vi "GUI Manual.vi"() -> ()   [LabVIEW 2019]
panel:
  in  "String 3":string="Блок управление ВБ"
  in  "String 2":string="Гидростанция очистки и охлаждения"
  in  "Tab Control 2":enum32{"Управление", "Настройки"}(tab)
  out "DI 31":bool caption="Релеле котроля фаз"
  out "Boolean Round 2":bool=TRUE
  out "DI 30":bool=TRUE caption="Высокая уровень\nпредупреждение"
  out "DI 29":bool=TRUE caption="Высокая температура\nавария"
  out "DI 28":bool caption="Низкая температура\nпредупреждение"
  out "DI 27":bool caption="Низкая температура\nавария"
  out "DI 26":bool caption="Высокий уровень\nпредупреждение"
  out "DI 25":bool caption="Высокий уровень\nавария"
  out "DI 24":bool=TRUE caption="Низкий уровень\nпредупреждение"
  out "DI 23":bool=TRUE caption="Низкий уровень\nавария"
  out "DI 22":bool caption="Ошибка \nвыключение"
  out "DI 21":bool caption="Ошибка \nвключение"
  out "DI 20":bool caption="Незапланированное \nвыключение"
  out "DI 19":bool caption="Незапланированное \nвключение"
  in  "Reset Button 2":bool
  in  "Close Button 3":bool
  in  "Start Button 2":bool
  in  "State 2":string="Отключенна" caption="State"
  out "Vertical Fill Indicator 2":dbl(slide)=5.954198473282443 caption="Температура масла" scale=0.0..100.0
  out "Уровень  масла 2":dbl(slide)=37.72455089820359 caption="Уровень  масла" scale=0.0..100.0
  out "DI 18":bool caption="Реле"
  out "DI 17":bool caption="Автомат"
  out "DI 16":bool caption="Контактор"
  in  "HIHI 8":dbl caption="HIHI"
  in  "HI 4":dbl caption="HI"
  in  "LOLO 4":dbl caption="LOLO"
  in  "LO 4":dbl caption="LO"
  in  "HIHI 7":dbl
  in  "HI 3":dbl
  in  "LOLO 3":dbl
  in  "LO 3":dbl
  in  "HIHI 6":dbl caption="Таймаут включения"
  in  "HIHI 5":dbl caption="Таймаут выключения"
  in  "OK Button 2":bool
  in  "Close Button 4":bool
  in  "String":string="Гидростанция очистки и охлаждения"
  in  "Tab Control":enum32{"Управление", "Настройки"}(tab)
  out "DI 15":bool caption="Релеле котроля фаз"
  out "Boolean Round":bool=TRUE
  out "DI 14":bool=TRUE caption="Высокая уровень\nпредупреждение"
  out "DI 13":bool=TRUE caption="Высокая температура\nавария"
  out "DI 12":bool caption="Низкая температура\nпредупреждение"
  out "DI 11":bool caption="Низкая температура\nавария"
  out "DI 10":bool caption="Высокий уровень\nпредупреждение"
  out "DI 9":bool caption="Высокий уровень\nавария"
  out "DI 8":bool=TRUE caption="Низкий уровень\nпредупреждение"
  out "DI 7":bool=TRUE caption="Низкий уровень\nавария"
  out "DI 6":bool caption="Ошибка \nвыключение"
  out "DI 5":bool caption="Ошибка \nвключение"
  out "DI 4":bool caption="Незапланированное \nвыключение"
  out "DI 3":bool caption="Незапланированное \nвключение"
  in  "Reset Button":bool
  in  "Close Button":bool
  in  "Start Button":bool
  in  "State":string="Отключенна"
  out "Vertical Fill Indicator":dbl(slide)=5.954198473282443 caption="Температура масла" scale=0.0..100.0
  out "Уровень  масла":dbl(slide)=37.72455089820359 scale=0.0..100.0
  out "DI 2":bool caption="Реле"
  out "DI 1":bool caption="Автомат"
  out "DI 0":bool caption="Контактор"
  in  "HIHI 2":dbl caption="HIHI"
  in  "HI 2":dbl caption="HI"
  in  "LOLO 2":dbl caption="LOLO"
  in  "LO 2":dbl caption="LO"
  in  "HIHI":dbl
  in  "HI":dbl
  in  "LOLO":dbl
  in  "LO":dbl
  in  "HIHI 3":dbl caption="Таймаут включения"
  in  "HIHI 4":dbl caption="Таймаут выключения"
  in  "OK Button":bool
  in  "Close Button 2":bool
  # "Насос перекачки в бак подачи"
  # "Уровень  масла"
  # "Температура масла"
  # "Оставить здесь или перенести в \nобщий конфиг"
  # "Уровень  масла"
  # "Температура масла"
  # "Оставить здесь или перенести в \nобщий конфиг"
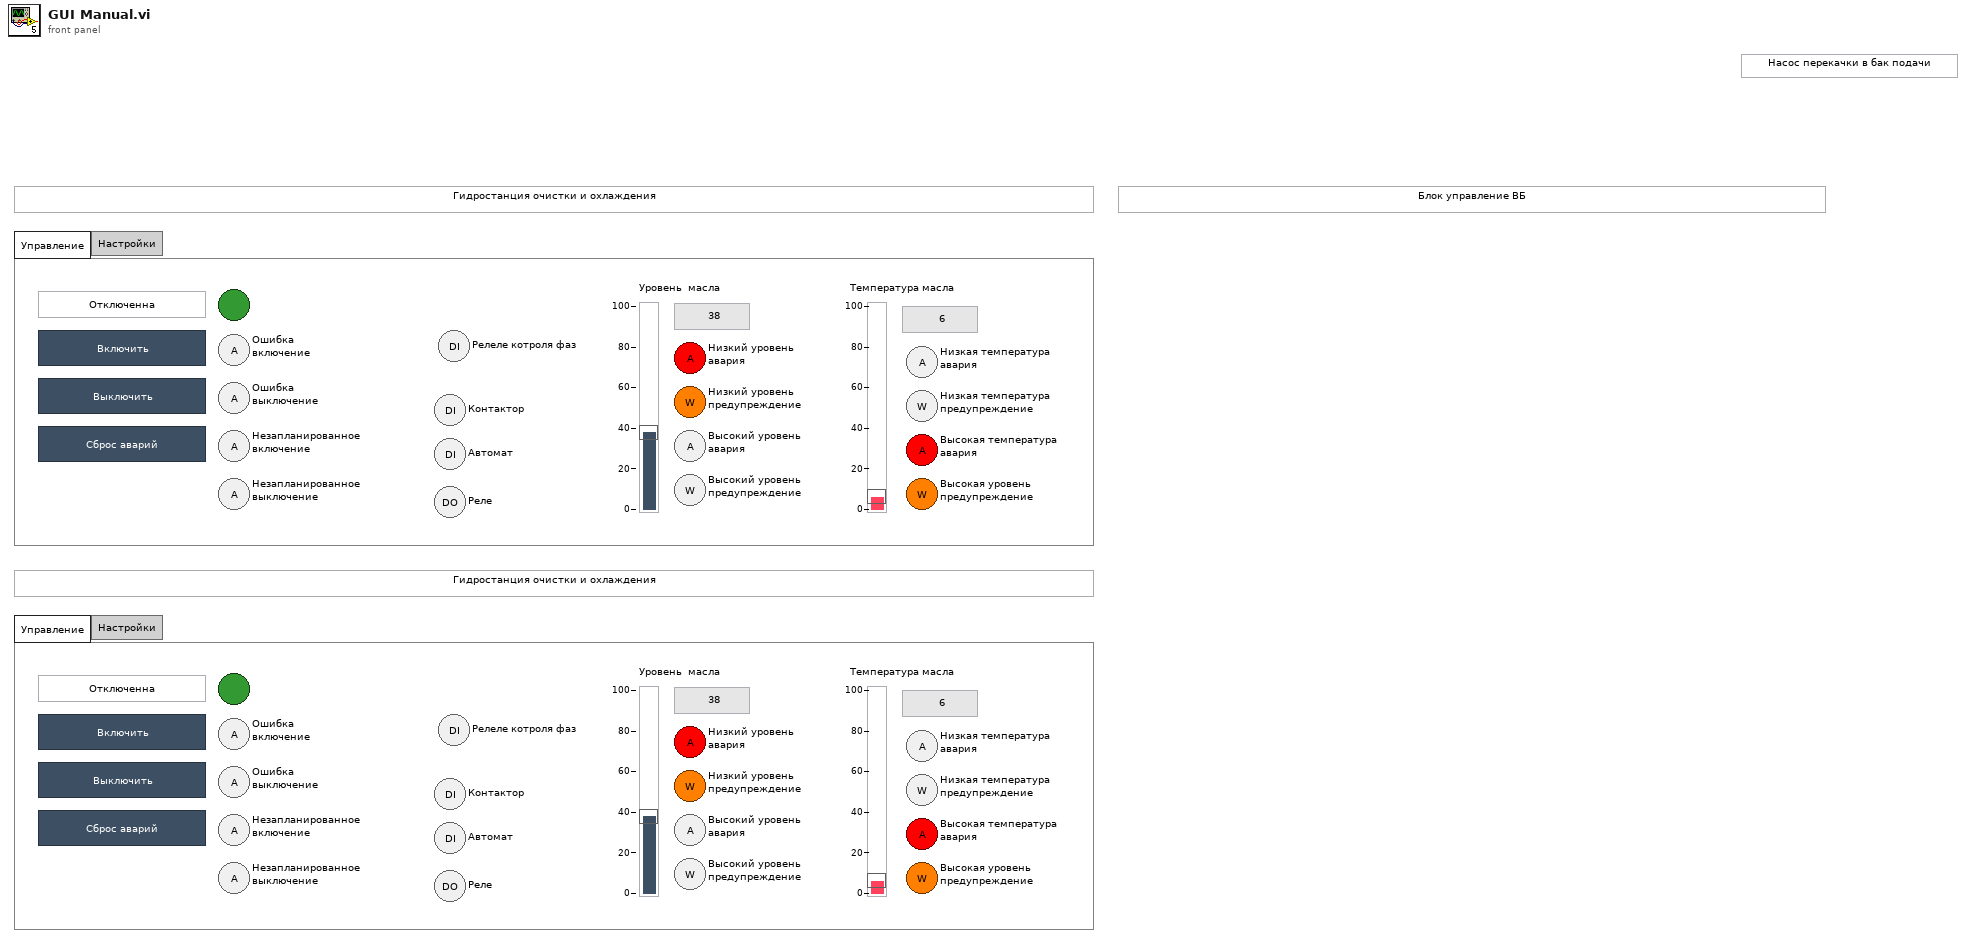
[diagram p1: front panel]
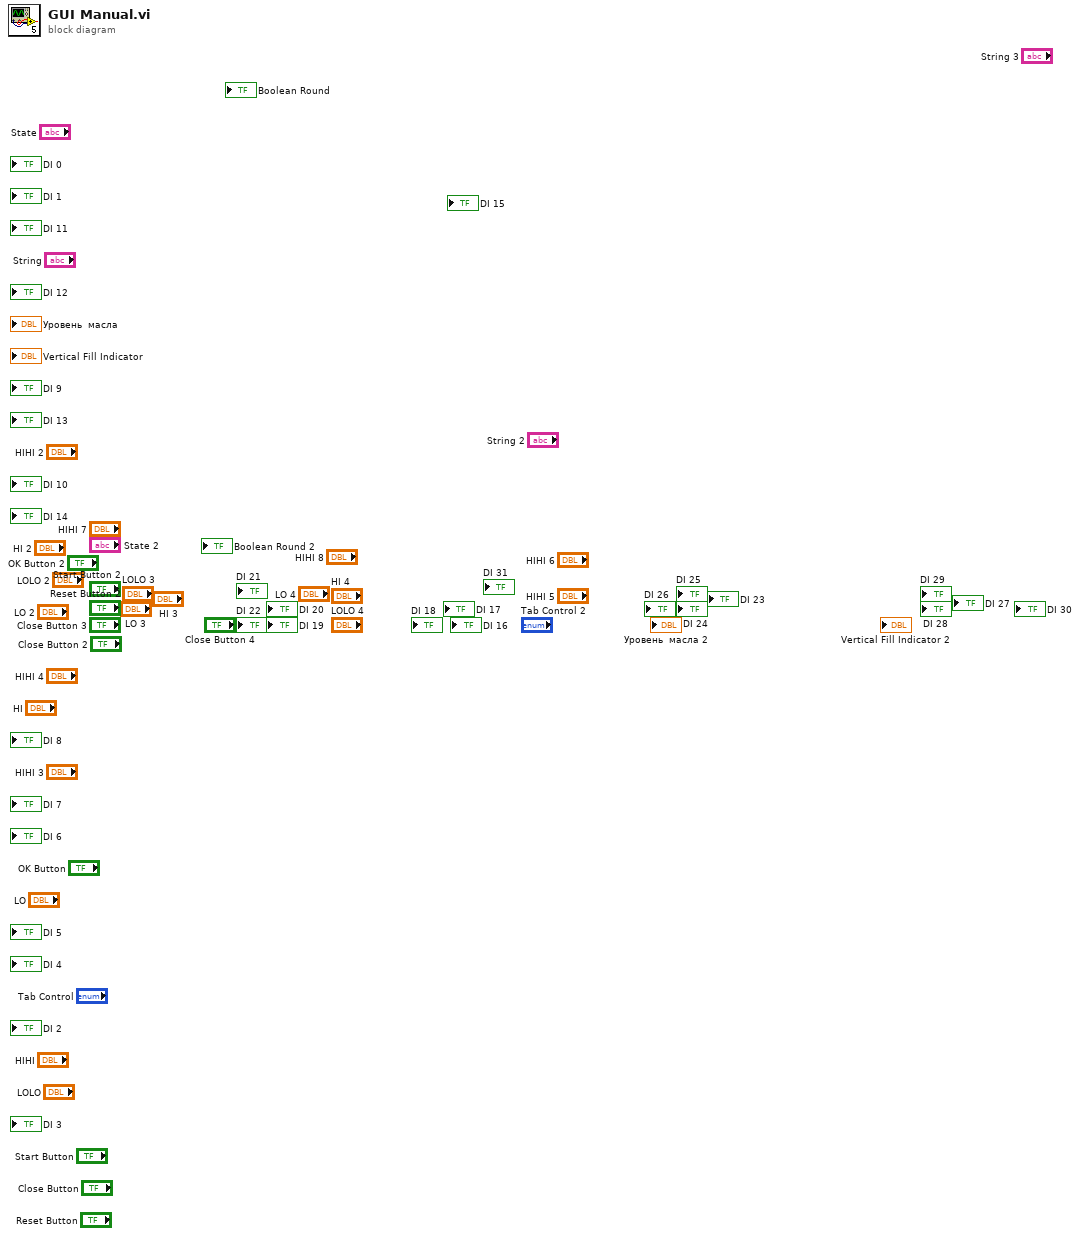
[diagram p0: block diagram]
diagram:
